vi "Piezo Message Loop new.vi"(8 "error in (no error)":errorcluster, 10 "Data Notifiers":T1, 11 "Message Queues":T2) -> (0 "error out":errorcluster)   [LabVIEW 2013, in "Piezo.lvlib"]
uses:
  Piezo.lvlib
  support/Message Queue/All Message Queues.ctl
  support/Message Queue/Message Cluster.ctl
  support/Data Notifiers/All Data Notifiers.ctl
  Acquisition/APD Notifier Cluster.ctl
  Piezo display.ctl
  XY/XY Display.ctl
  Capacitive/Capacitive Signal Cluster.ctl
  Feedback/Error Signal.ctl
  Piezo State.ctl
  Hardware Configuration Piezo.ctl
  support/Message Queue/Enqueue Message (Single).vi
  <vilib>/Utility/error.llb/Error Cluster From Error Code.vi
  <vilib>/ErrorRing/Error Ring.xnode
  support/Message Queue/Message Queue.lvlib
  Acquisition/Acquisition.lvlib
  XY/XY.lvlib
  support/Data Notifiers/Data Notifiers.lvlib
  Capacitive/Capacitive.lvlib
  Feedback/Feedback.lvlib
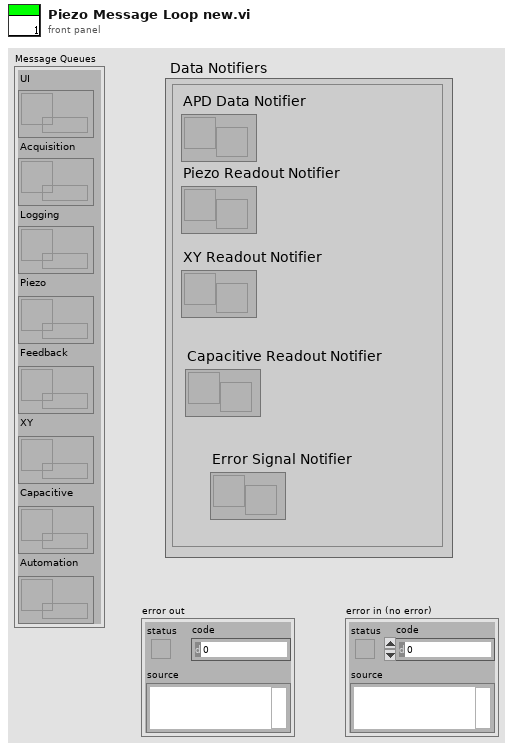
[diagram p1: front panel]
types:
  T1 = typedef "Data Notifiers.lvlib/All Data Notifiers.ctl" = cluster{"APD Data Notifier":refnum<notifier>, "Piezo Readout Notifier":refnum<notifier>, "XY Readout Notifier":refnum<notifier>, "Capacitive Readout Notifier":refnum<notifier>, "Error Signal Notifier":refnum<notifier>}
  T2 = typedef "Message Queue.lvlib/All Message Queues.ctl" = cluster{"UI":refnum<queue>, "Acquisition":refnum<queue>, "Logging":refnum<queue>, "Piezo":refnum<queue>, "Feedback":refnum<queue>, "XY":refnum<queue>, "Capacitive":refnum<queue>, "Automation":refnum<queue>}
  T3 = typedef "Piezo.lvlib/Hardware Configuration Piezo.ctl" = cluster{"DAQmx Channel":tag, "Max Input":dbl, "Min Input":dbl, "Samples per ch.":dbl, "Setpoint (um)":dbl, "DAQmx Task":refnum<k21>}
  T4 = typedef "Piezo.lvlib/Piezo State.ctl" = enum16{"Idle", "Acquiring"}
  T5 = typedef "Acquisition.lvlib/APD Notifier Cluster.ctl" = cluster{"data":dbl[][], "t0":i32}
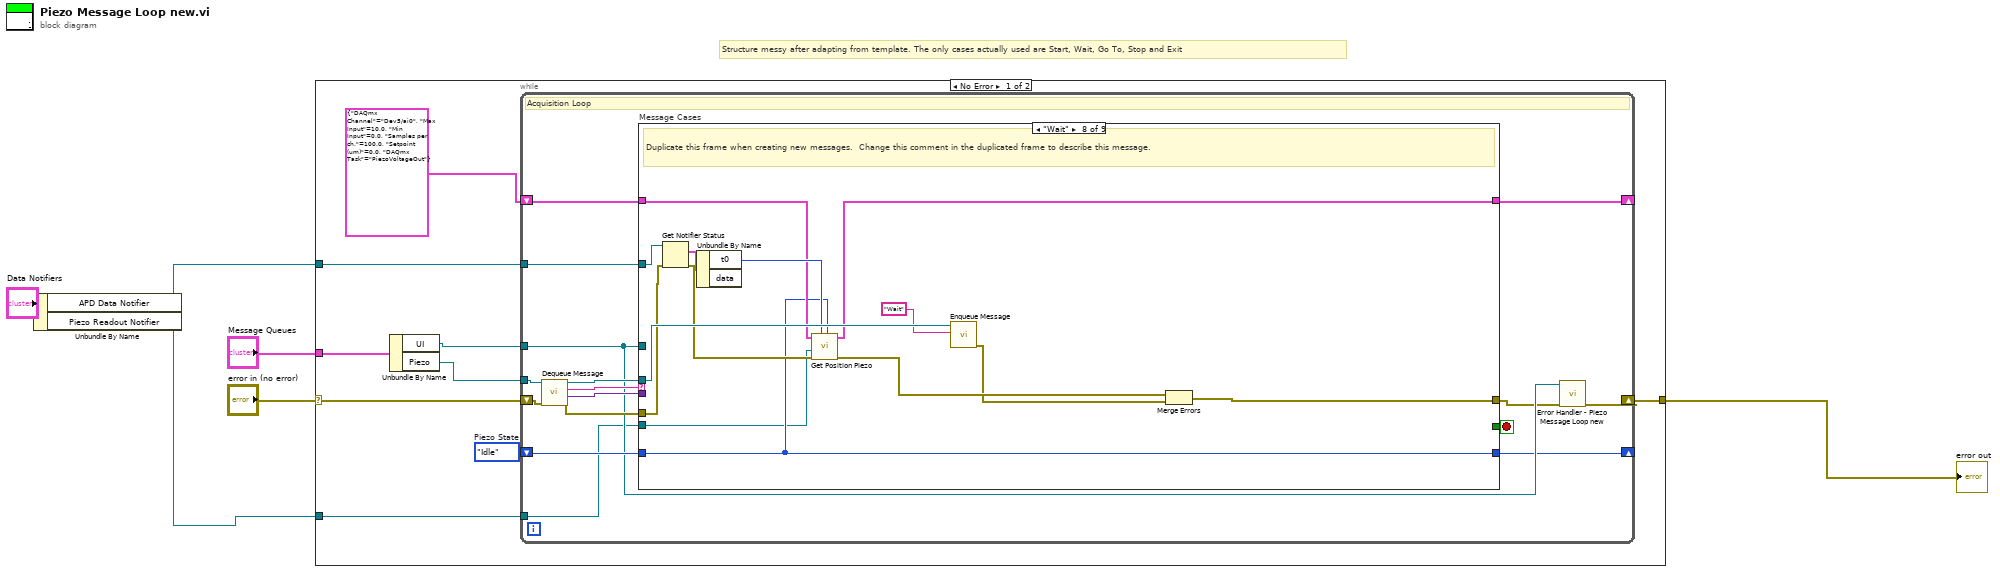
[diagram p0: block diagram]
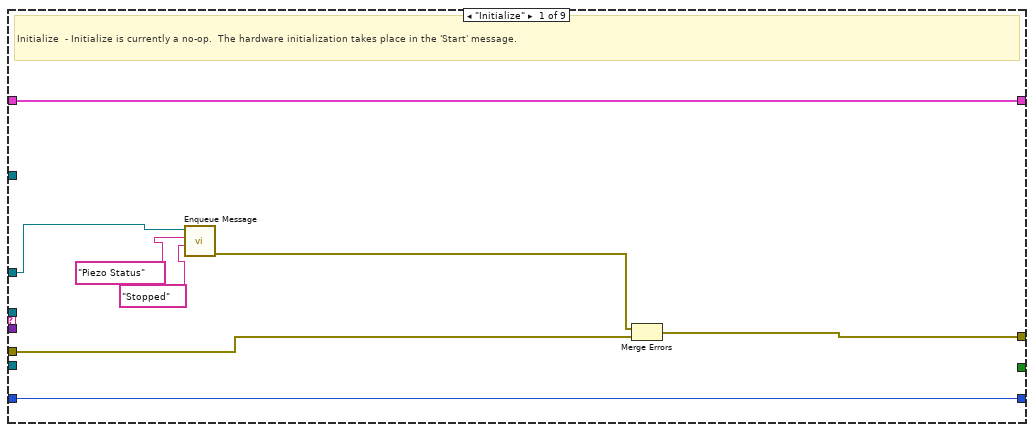
[diagram p2: hidden frame]
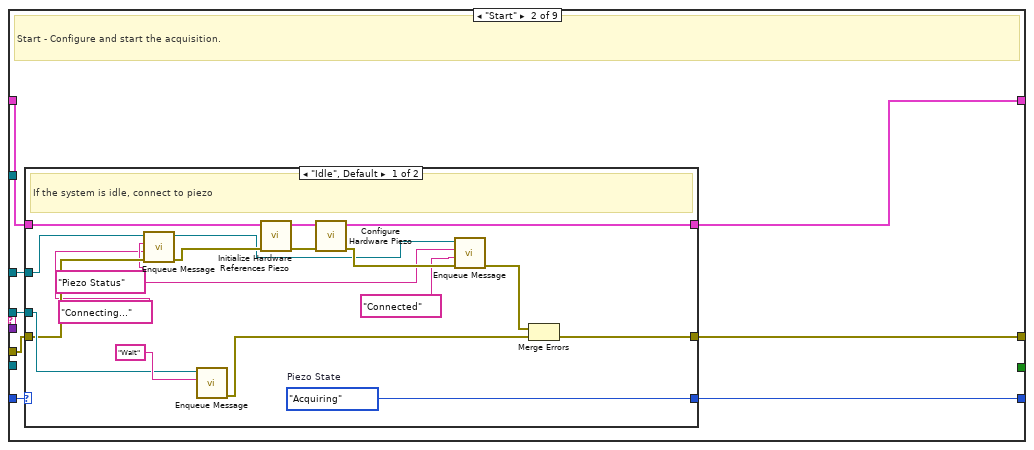
[diagram p3: hidden frame]
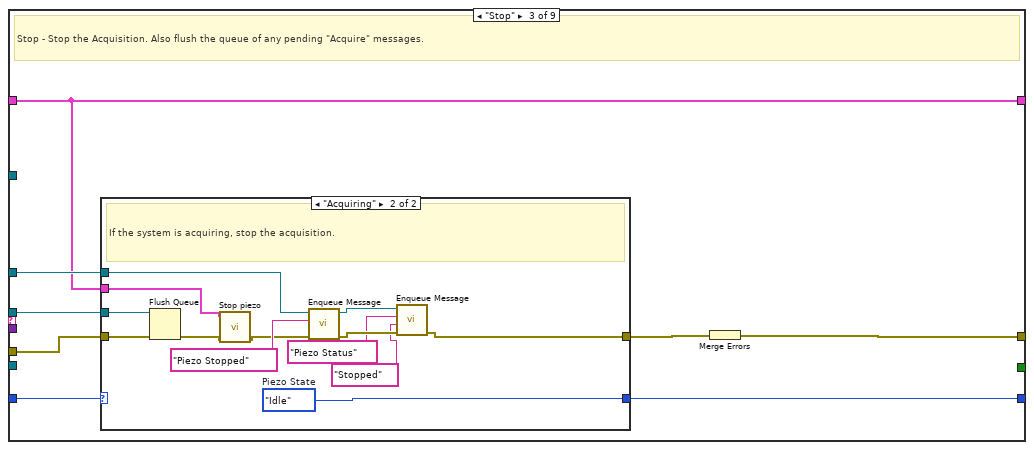
[diagram p5: hidden frame]
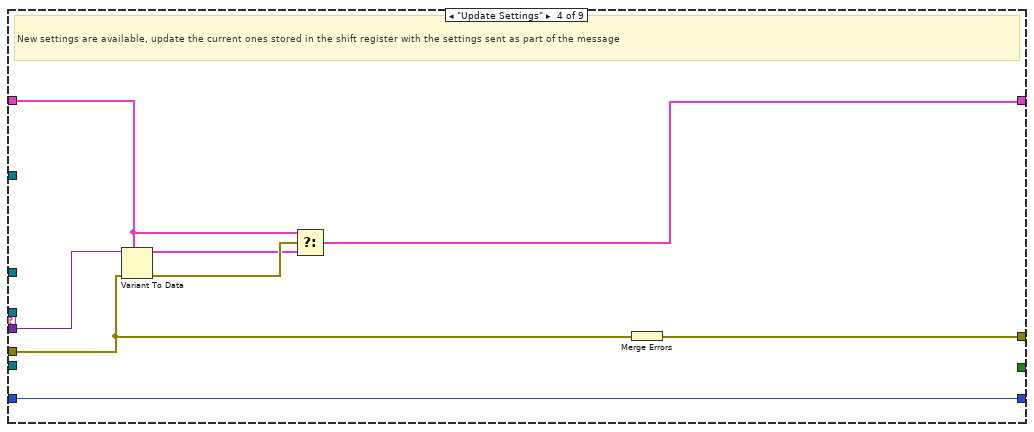
[diagram p7: hidden frame]
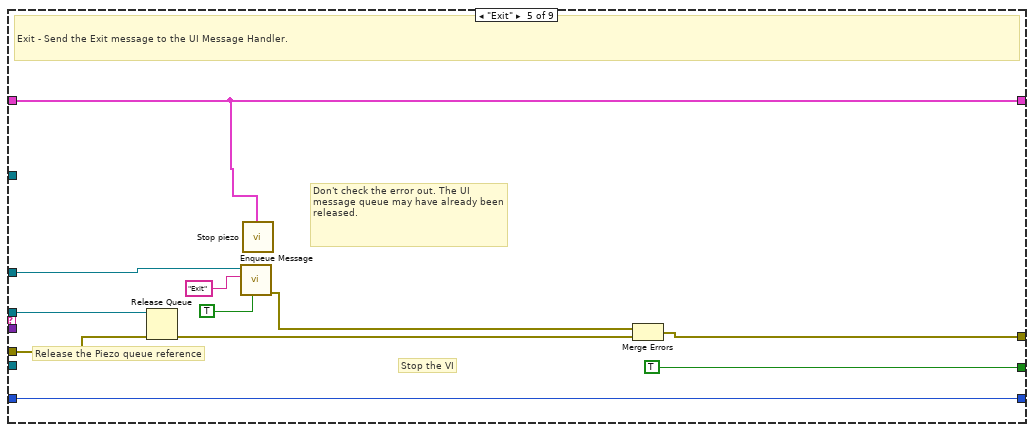
[diagram p8: hidden frame]
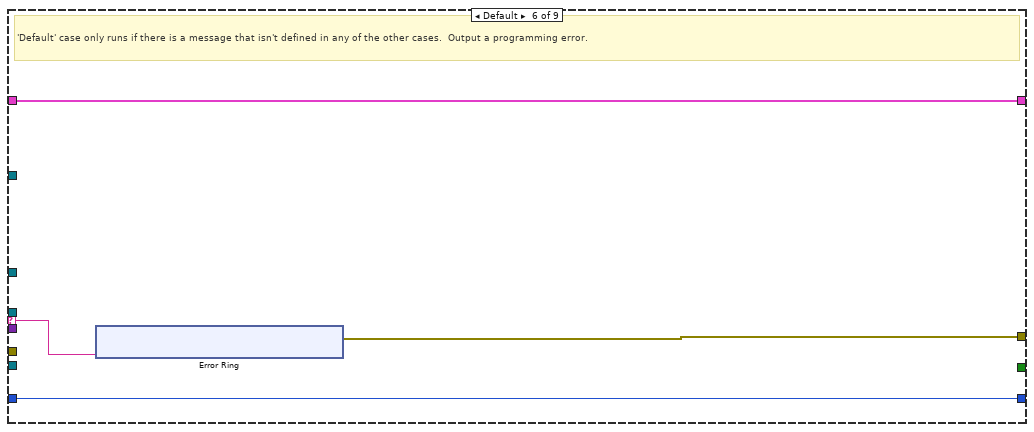
[diagram p9: hidden frame]
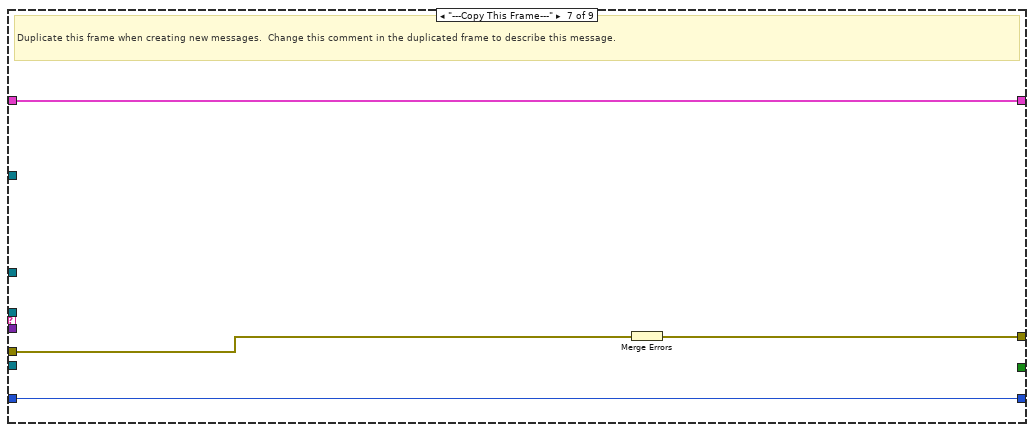
[diagram p10: hidden frame]
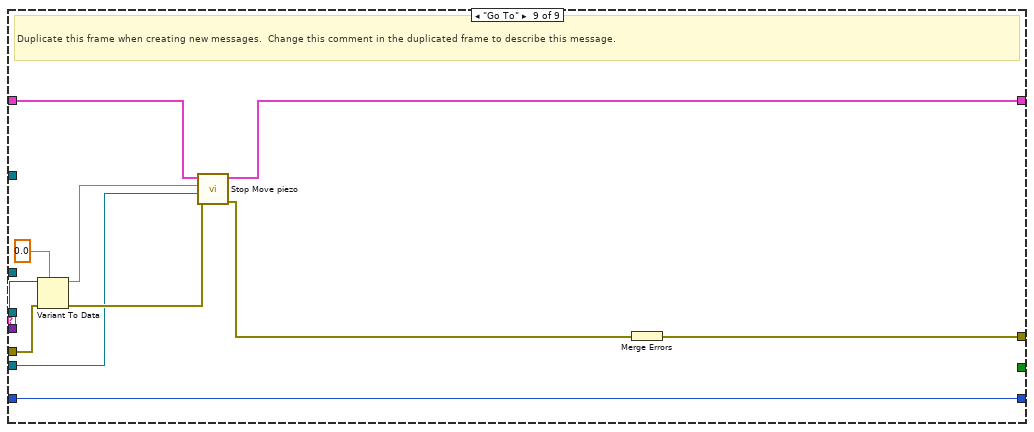
[diagram p11: hidden frame]
diagram:
  # "Structure messy after adapting from template. The only cases actually used are Start, Wait, Go To, Stop and Exit"
  n1 = Unbundle By Name("Data Notifiers") -> ("APD Data Notifier"=w2:refnum<notifier>, "Piezo Readout Notifier"=w1:refnum<notifier>)
  n2 = case shown="No Error" "error in (no error)" {
    selector: "error in (no error)" -> [w10 w151]
    tunnel: "Message Queues" -> [w15 _]
    tunnel: [w13 w151] -> w5
    tunnel: w1 -> [w9 _]
    tunnel: w2 -> [w8 _]
    frame No Error {
      w11 = Piezo_State."Idle"  # Piezo State
      n3 = Unbundle By Name(w15) -> ("UI"=w12:refnum<queue>, "Piezo"=w14:refnum<queue>)
      n4 = while {
        tunnel: w14 -> [w24]
        shift-right: [w19] -> _
        shift-left: T3 {"DAQmx Channel"="Dev5/ai0", "Max Input"=10.0, "Min Input"=0.0, "Samples per ch."=100.0, "Setpoint (um)"=0.0, "DAQmx Task"="PiezoVoltageOut"} ("Hardware Configuration") -> [w31]
        shift-right: [w21] -> w13
        shift-left: w10 -> [w29]
        tunnel: w12 -> [w22]
        shift-right: [w20] -> _
        shift-left: w11 -> [w23]
        tunnel: w9 -> [w17]
        tunnel: w8 -> [w16]
        stop <- w30 stop-if-true
        # "Acquisition Loop"
        n5 = call "Dequeue Message.vi"("error in (no error)"=w29, "Message Queue"=w24) -> ("error out"=w28:errorcluster, "Message Data"=w26:variant, "Message"=w27:string, "dup Message Queue"=w25:refnum<queue>)  [unwired: 6 in]
        n6 = case "Message Cases" shown="\"Wait\"" w27 {
          selector: w27 -> [_ _ _ _ _ w114 _ _ _]
          tunnel: w25 -> [_ w44 w74 _ w106 _ _ w137 _]
          tunnel: w28 -> [w38 w45 w75 w94 w108 _ w125 w133 w146]
          tunnel: [w39 w47 w76 w99 w109 w113 w124 w139 w150] -> w18
          tunnel: w31 -> [w36 w46 w69 w95 w104 w111 w122 w129 w145]
          tunnel: [_ _ _ _ TRUE _ _ _ _] -> w30
          tunnel: w26 -> [_ _ _ w98 _ _ _ _ w148]
          tunnel: w22 -> [w34 w40 w73 _ w101 _ _ _ _]
          tunnel: w23 -> [w37 w43 w72 w93 w105 w112 w123 w127 w149]
          tunnel: [w37 w42 w71 w93 w105 w112 w123 w127 w149] -> w20
          tunnel: [w36 w41 w69 w92 w104 w111 w122 w128 w144] -> w19
          tunnel: w17 -> [_ _ _ _ _ _ _ w126 w141]
          tunnel: w16 -> [_ _ _ _ _ _ _ w132 _]
          frame "Initialize" {
            # "Initialize  - Initialize is currently a no-op.  The hardware initialization takes place in the 'Start' message."
            n7 = call-poly "Enqueue Message.vi"("Message Data"="Stopped" ("Message"), "Message"="Piezo Status", "Message Queue"=w34) -> ("error out"=w33:errorcluster)  [unwired: 7 in, 1 out]
            n8 = Merge Errors(w33, w38) -> (w39:errorcluster)
          }
          frame "Start" {
            # "Start - Configure and start the acquisition."
            n9 = case shown="\"Idle\", Default" w43 {
              selector: w43 -> [_ w66]
              tunnel: [w65 w68] -> w47
              tunnel: w46 -> [w64 w67]
              tunnel: w45 -> [w52 w68]
              tunnel: w44 -> [w58 _]
              tunnel: [w61 w67] -> w41
              tunnel: [w60 w66] -> w42
              tunnel: w40 -> [w53 _]
              frame "Idle", Default {
                w49 = "Piezo Status" ("Message")
                w60 = Piezo_State."Acquiring"  # Piezo State
                # "If the system is idle, connect to piezo"
                n10 = call-poly "Enqueue Message.vi"("error in (no error)"=w52, "Message Data"="Connecting..." ("Message"), "Message"=w49, "Message Queue"=w53) -> ("error out"=w51:errorcluster, "dup Message Queue"=w50:refnum<queue>)  [unwired: 6 in]
                n11 = call-poly "Enqueue Message.vi"("Message"="Wait", "Message Queue"=w58) -> ("error out"=w57:errorcluster)  [unwired: 8 in, 1 out]
                n12 = call "Initialize Hardware References Piezo.vi"("error in (no error)"=w51, "Hardware Configuration"=w64) -> ("error out"=w63:errorcluster, "Hardware Configuration 2"=w62:T3)  [unwired: 8 in]
                n13 = call "Configure Hardware Piezo.vi"("error in (no error)"=w63, "Hardware Configuration in"=w62) -> ("error out"=w56:errorcluster, "Hardware Configuration out"=w61:T3)  [unwired: 8 in]
                n14 = call-poly "Enqueue Message.vi"("error in (no error)"=w56, "Message Data"="Connected" ("Message"), "Message"=w49, "Message Queue"=w50) -> ("error out"=w55:errorcluster)  [unwired: 6 in, 1 out]
                n15 = Merge Errors(w55, w57) -> (w65:errorcluster)
              }
              frame "Acquiring" {
                # "The system is already acquiring. Ignore the \"Start\" message."
              }
            }
          }
          frame "Stop" {
            # "Stop - Stop the Acquisition. Also flush the queue of any pending \"Acquire\" messages."
            n16 = case shown="\"Acquiring\"" w72 {
              selector: w72 -> [w78 _]
              tunnel: w75 -> [w77 w91]
              tunnel: w69 -> [_ w87]
              tunnel: w74 -> [_ w90]
              tunnel: w73 -> [_ w89]
              tunnel: [w78 w84] -> w71
              tunnel: [w77 w81] -> w70
              frame "Idle", Default {
                # "The system is already idle. Ignore the \"Stop\" message."
              }
              frame "Acquiring" {
                w84 = Piezo_State."Idle"  # Piezo State
                # "If the system is acquiring, stop the acquisition."
                n17 = Flush Queue(queue=w90, error in (no error)=w91) -> (error out=w86:errorcluster)  [unwired: 2 out]
                n18 = call "Stop piezo.vi"("error in (no error)"=w86, "Hardware Configuration"=w87) -> ("error out"=w85:errorcluster)  [unwired: 9 in]
                n19 = call-poly "Enqueue Message.vi"("error in (no error)"=w85, "Message"="Piezo Stopped", "Message Queue"=w89) -> ("error out"=w82:errorcluster, "dup Message Queue"=w83:refnum<queue>)  [unwired: 7 in]
                n20 = call-poly "Enqueue Message.vi"("error in (no error)"=w82, "Message Data"="Stopped" ("Message"), "Message"="Piezo Status", "Message Queue"=w83) -> ("error out"=w81:errorcluster)  [unwired: 6 in, 1 out]
              }
            }
            n21 = Merge Errors(w70) -> (w76:errorcluster)
          }
          frame "Update Settings" {
            # "New settings are available, update the current ones stored in the shift register with the settings sent as part of the message"
            n22 = Variant To Data(error in=w94, type=w95, Variant=w98) -> (data=w96:T3, error out=w97:errorcluster)
            n23 = Select(t=w95, s=w97, f=w96) -> (s? t:f=w92:T3)
            n24 = Merge Errors(w94) -> (w99:errorcluster)
          }
          frame "Exit" {
            # "Don't check the error out. The UI message queue may have already been released."
            # "Release the Piezo queue reference"
            # "Stop the VI"
            # "Exit - Send the Exit message to the UI Message Handler."
            n25 = Release Queue(queue=w106, error in (no error)=w108) -> (error out=w107:errorcluster)  [unwired: 1 in, 2 out]
            n26 = call-poly "Enqueue Message.vi"("Priority Message? (F)"=TRUE, "Message"="Exit", "Message Queue"=w101) -> ("error out"=w100:errorcluster)  [unwired: 7 in, 1 out]
            n27 = call "Stop piezo.vi"("Hardware Configuration"=w104) -> ()  [unwired: 10 in, 1 out]
            n28 = Merge Errors(w100, w107) -> (w109:errorcluster)
          }
          frame Default {
            # "'Default' case only runs if there is a message that isn't defined in any of the other cases.  Output a programming error."
            n29 = xnode "Error Ring"("parameter 0"=w114) -> ("error out"=w113:errorcluster)
          }
          frame "---Copy This Frame---" {
            # "Duplicate this frame when creating new messages.  Change this comment in the duplicated frame to describe this message."
            n30 = Merge Errors(w125) -> (w124:errorcluster)
          }
          frame "Wait" {
            # "Duplicate this frame when creating new messages.  Change this comment in the duplicated frame to describe this message."
            n31 = Get Notifier Status(notifier=w132, error in (no error)=w133) -> (current notification=w131:T5, error out=w134:errorcluster)  [unwired: 3 out]
            n32 = Unbundle By Name(w131) -> ("t0"=w130:i32)  [unwired: 1 out]
            n33 = call "Get Position Piezo.vi"("Piezo State"=w127, "Counter Time"=w130, "error in (no error)"=w134, "notifier out"=w126, "Hardware Configuration"=w129) -> ("error out"=w138:errorcluster, "Hardware Configuration 2"=w128:T3)  [unwired: 2 in, 3 out]
            n34 = call-poly "Enqueue Message.vi"("Message"="Wait", "Message Queue"=w137) -> ("error out"=w135:errorcluster)  [unwired: 8 in, 1 out]
            n35 = Merge Errors(w138, w135) -> (w139:errorcluster)
          }
          frame "Go To" {
            # "Duplicate this frame when creating new messages.  Change this comment in the duplicated frame to describe this message."
            n36 = Variant To Data(error in=w146, type=sgl 0.0, Variant=w148) -> (data=w143:sgl, error out=w142:errorcluster)
            n37 = call "Stop Move piezo.vi"("error in (no error)"=w142, "notifier out"=w141, "MOVE TO [MICRON]"=w143, "Hardware Configuration in"=w145) -> ("error out"=w140:errorcluster, "Hardware Configuration out"=w144:T3)  [unwired: 6 in]
            n38 = Merge Errors(w140) -> (w150:errorcluster)
          }
        }
        n39 = call "Error Handler - Piezo Message Loop new.vi"("error in (no error)"=w18, "Message Queue"=w22) -> ("dup error in"=w21:errorcluster)  [unwired: 8 in, 1 out]
      }
    }
    frame Error {
    }
  }
  "error out" <- w5
